vi "fromDevVarStringArray.vi"(1 "argin":string[](array[string])) -> (0 "ArgIO":cluster{"num data":u8[], "str data":string[]})   [LabVIEW 2014, in "tango.lvlib"]
uses:
  tango.lvlib
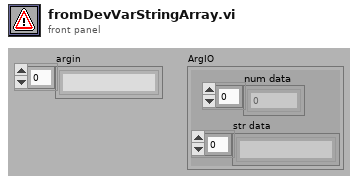
[diagram p1: front panel]
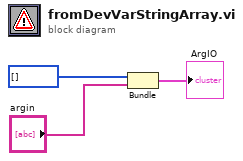
[diagram p0: block diagram]
diagram:
  n1 = Bundle(u8[] [], "argin"="argin") -> (→"ArgIO":cluster{u8[], "argin":string[]})  [unwired: 1 in]
